vi "Sort Unhandled Errors By Error Code Ascending.vi"(1 "Unhandled Errors (unsorted)":T1[](array[typedef])) -> (0 "Unhandled Errors (sorted by error code, ascending)":T1[](array[typedef]))   [LabVIEW 2016, in "Error Manager.lvlib"]
doc: "This VI takes as input an array of unsorted Unhandled Errors, and outputs an array of Unhandled Errors sorted by error code, in ascending order (smallest, or most negative error codes first).\n\nThe sorting algorithm is a form of Selection Sort. Selection Sort is not the most efficient sorting algorithm (for example Merge Sort is more efficient), but it's one of the easiest sorting algorithms to implement and understand.\n\nIn practice, it is expected that the 'Unhandled Errors (unsorted)' input array to contain 1 element most of the times (therefore no sorting required), and up to a few (say up to 5) elements at a maximum. So computational efficiency is not that important due to the small input size."
uses:
  Error Manager.lvlib
  Unhandled Error (cluster).ctl
panel:
  # "Input\nInputs to the VI"
  # "Development\nControls or indicators that are useful for development or testing, but which are not outputs of the VI."
  # "Output\nOutputs of the VI"
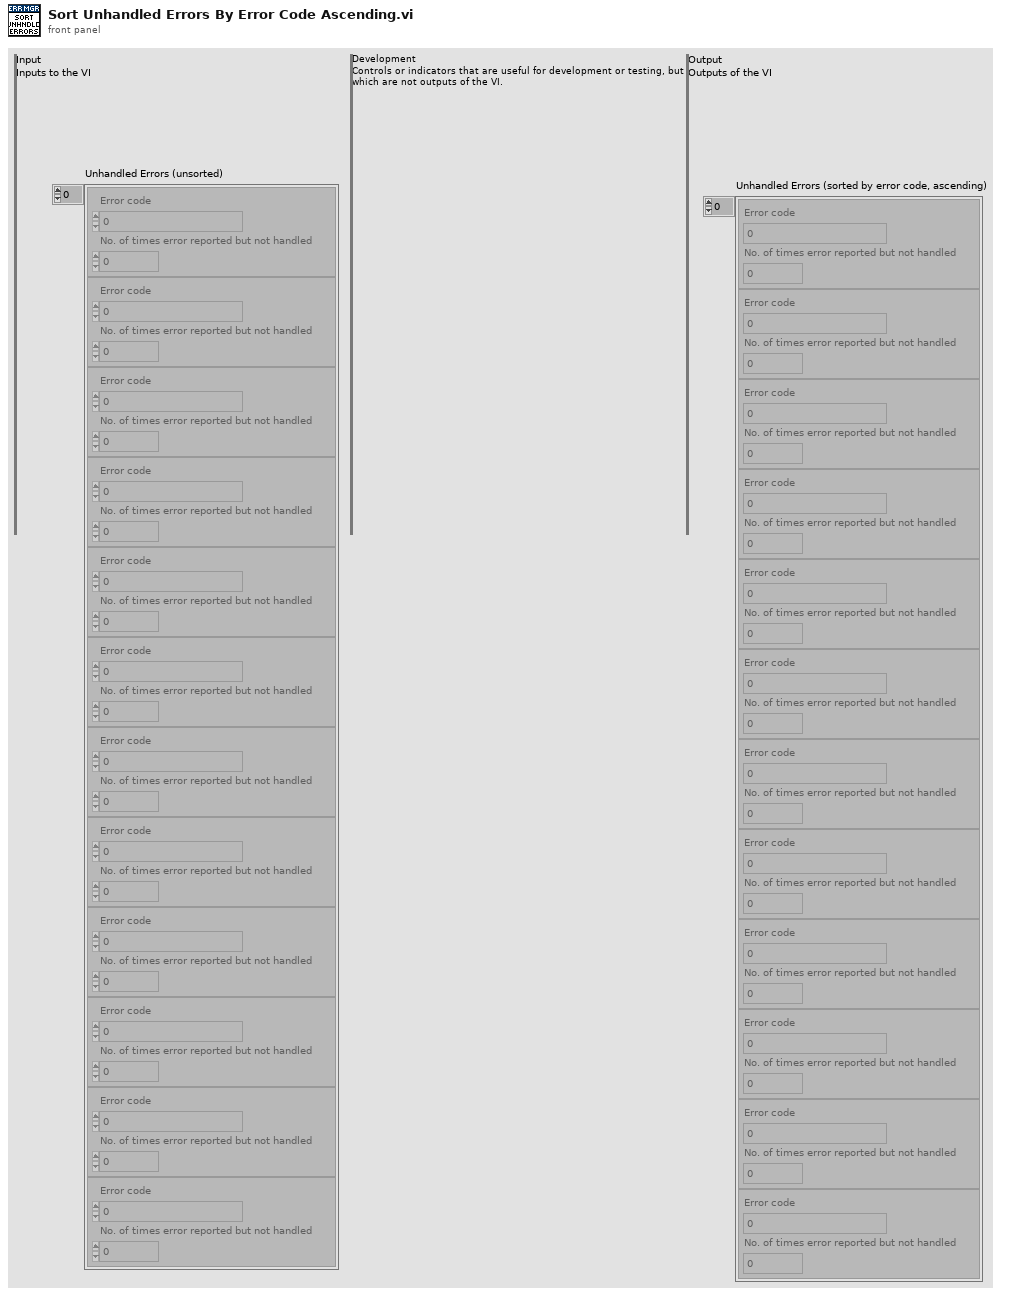
[diagram p1: front panel]
types:
  T1 = typedef "Error Manager.lvlib/Unhandled Error (cluster).ctl" = cluster{"Error code":i32, "No. of times error reported but not handled":u32}
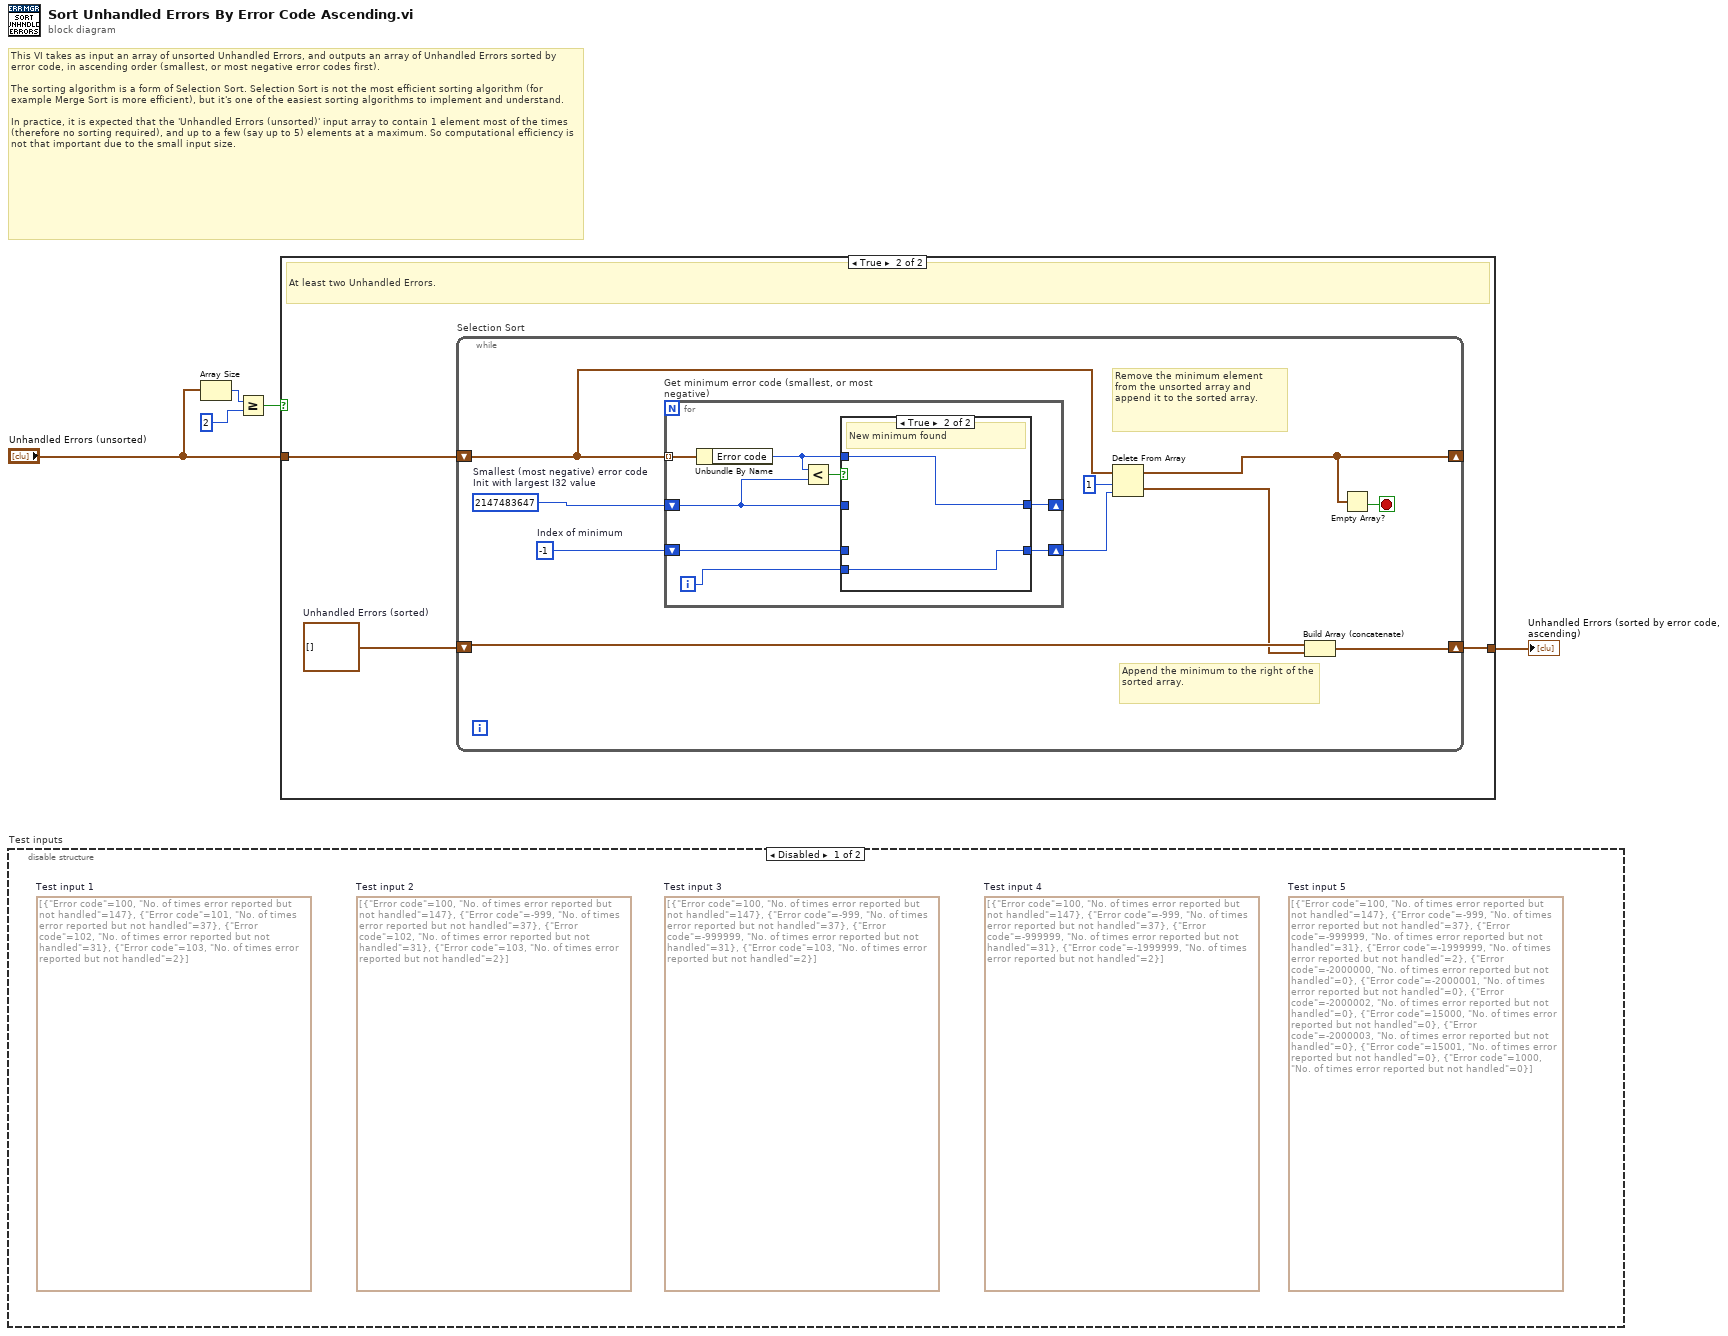
[diagram p0: block diagram]
diagram:
  # "This VI takes as input an array of unsorted Unhandled Errors, and outputs an array of Unhandled Errors sorted by error code, in ascending order (smallest, or most negative error codes first).\n\nThe sorting algorithm is a form of Selection Sort. Selection Sort is not the most efficient sorting algorithm (for example Merge Sort is more efficient), but it's one of the easiest sorting algorithms to implement and understand.\n\nIn practice, it is expected that the 'Unhandled Errors (unsorted)' input array to contain 1 element most of the times (therefore no sorting required), and up to a few (say up to 5) elements at a maximum. So computational efficiency is not that important due to the small input size."
  n1 = disable-structure "Test inputs" shown="Disabled" {
    frame Disabled {
      (unwired) T1[] [{"Error code"=100, "No. of times error reported but not handled"=147}, {"Error code"=-999, "No. of times error reported but not handled"=37}, {"Error code"=-999999, "No. of times error reported but not handled"=31}, {"Error code"=-1999999, "No. of times error reported but not handled"=2}, {"Error code"=-2000000, "No. of times error reported but not handled"=0}, {"Error code"=-2000001, "No. of times error reported but not handled"=0}, {"Error code"=-2000002, "No. of times error reported but not handled"=0}, {"Error code"=15000, "No. of times error reported but not handled"=0}, {"Error code"=-2000003, "No. of times error reported but not handled"=0}, {"Error code"=15001, "No. of times error reported but not handled"=0}, {"Error code"=1000, "No. of times error reported but not handled"=0}]  # Test input 5
      (unwired) T1[] [{"Error code"=100, "No. of times error reported but not handled"=147}, {"Error code"=-999, "No. of times error reported but not handled"=37}, {"Error code"=-999999, "No. of times error reported but not handled"=31}, {"Error code"=-1999999, "No. of times error reported but not handled"=2}]  # Test input 4
      (unwired) T1[] [{"Error code"=100, "No. of times error reported but not handled"=147}, {"Error code"=-999, "No. of times error reported but not handled"=37}, {"Error code"=-999999, "No. of times error reported but not handled"=31}, {"Error code"=103, "No. of times error reported but not handled"=2}]  # Test input 3
      (unwired) T1[] [{"Error code"=100, "No. of times error reported but not handled"=147}, {"Error code"=-999, "No. of times error reported but not handled"=37}, {"Error code"=102, "No. of times error reported but not handled"=31}, {"Error code"=103, "No. of times error reported but not handled"=2}]  # Test input 2
      (unwired) T1[] [{"Error code"=100, "No. of times error reported but not handled"=147}, {"Error code"=101, "No. of times error reported but not handled"=37}, {"Error code"=102, "No. of times error reported but not handled"=31}, {"Error code"=103, "No. of times error reported but not handled"=2}]  # Test input 1
    }
    frame Enabled {
    }
  }
  n2 = Array Size(array="Unhandled Errors (unsorted)") -> (size(s)=w4:i32)
  n3 = Greater Or Equal?(x=w4, y=2) -> (x >= y?=w3:bool)
  n4 = case shown="True" w3 {
    tunnel: "Unhandled Errors (unsorted)" -> [w6 w9]
    tunnel: [w6 w7] -> w1
    frame False {
      # "0 or 1 Unhandled Errors. Nothing to sort."
    }
    frame True {
      w8 = T1[] []  # Unhandled Errors (sorted)
      # "At least two Unhandled Errors."
      n5 = while "Selection Sort" {
        shift-right: [w12] -> w7
        shift-left: w8 -> [w14]
        shift-right: [w11] -> _
        shift-left: w9 -> [w17]
        stop <- w10 stop-if-true
        w18 = -1  # Index of minimum
        w19 = 2147483647  # Smallest (most negative) error code Init with largest I32 value
        # "Remove the minimum element from the unsorted array and append it to the sorted array."
        # "Append the minimum to the right of the sorted array."
        n6 = for "Get minimum error code (smallest, or most negative)" {
          tunnel: w17 -> [w27] mode=indexing
          shift-right: [w24] -> _
          shift-left: w19 -> [w23]
          shift-right: [w22] -> w16
          shift-left: w18 -> [w20]
          i -> [w21]
          n7 = Unbundle By Name(w27) -> ("Error code"=w25:i32)
          n8 = Less?(x=w25, y=w23) -> (x < y?=w26:bool)
          n9 = case shown="True" w26 {
            tunnel: w25 -> [_ w31]
            tunnel: [w29 w31] -> w24
            tunnel: w23 -> [w29 _]
            tunnel: [w28 w30] -> w22
            tunnel: w21 -> [_ w30]
            tunnel: w20 -> [w28 _]
            frame False {
              # "Not a new minimum"
            }
            frame True {
              # "New minimum found"
            }
          }
        }
        n10 = Delete From Array "Delete From Array"(array=w17, length=1, index=w16) -> (deleted portion=w13:T1[], array with subset deleted=w11:T1[])
        n11 = Build Array (concatenate)(w14, w13) -> (w12:T1[])
        n12 = Empty Array?(array=w11) -> (empty?=w10:bool)
      }
    }
  }
  "Unhandled Errors (sorted by error code, ascending)" <- w1
